vi "Add Item to JSON String.vi"(10 "JSON String In":string, 11 "Customer DAO JSON in":refnum<class "Object DAO JSON.lvclass">) -> (2 "JSON string out":string, 3 "Customer DAO JSON out":refnum<class "Object DAO JSON.lvclass">)   [LabVIEW 2020, in "Object DAO JSON.lvclass"]
doc: "Converts cluster to a JSON string and adds it to the JSON object List."
uses:
  Object DAO JSON.lvclass
  C:/Users/fflores/Desktop/DataBase - Copy - Copy/Object DAO/Object DAO.lvclass
  Object DAO/Object DAO.lvclass/Object DAO.ctl
  Object DAO/Member Accessors/Get Object Information.vi
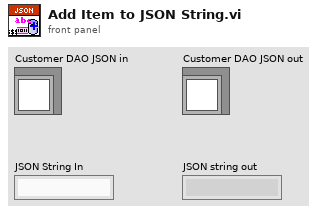
[diagram p1: front panel]
types:
  T1 = typedef "Object DAO.lvclass/Object Information.ctl" = cluster{"String":string, "Boolean":bool, "Numeric":dbl, "id":string}
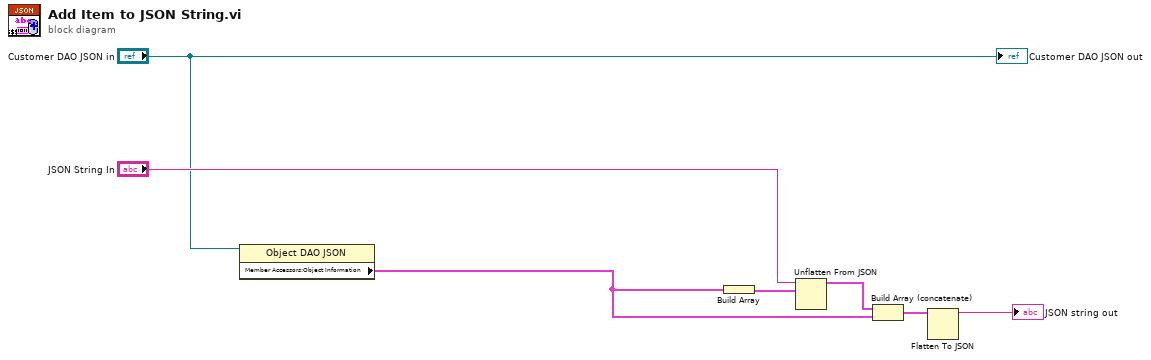
[diagram p0: block diagram]
diagram:
  n1 = property class="Object DAO JSON"(reference="Customer DAO JSON in") -> ("Member Accessors:Object Information"=w1:T1)  [unwired: 1 in, 2 out]
  n2 = Build Array(w1) -> (w5:T1[])
  n3 = Unflatten From JSON(JSON string="JSON String In", type and defaults=w5) -> (value=w6:T1[])  [unwired: 5 in, 1 out]
  n4 = Build Array (concatenate)(w6, w1) -> (w4:T1[])
  n5 = Flatten To JSON(anything=w4) -> (JSON string=→"JSON string out":string)  [unwired: 2 in, 1 out]
  "Customer DAO JSON out" <- "Customer DAO JSON in"
